vi "cwlaserShutterOpenClose.vi"(1 "mode":u16(ring) items=["close", "open"], 2 "wavelength (nm)":dbl) -> (0 "success":bool)   [LabVIEW 2017]
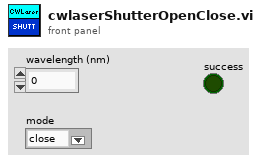
[diagram p1: front panel]
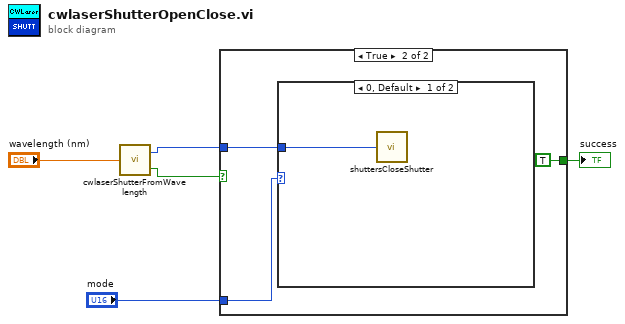
[diagram p0: block diagram]
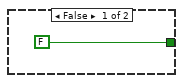
[diagram p2: hidden frame]
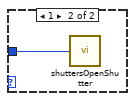
[diagram p3: hidden frame]
diagram:
  n1 = call "cwlaserShutterFromWavelength.vi"("wavelength (nm)"="wavelength (nm)") -> ("shutter"=w3:i32, "found"=w2:bool)
  n2 = case shown="True" w2 {
    tunnel: w3 -> [_ w8]
    tunnel: "mode" -> [_ w9]
    tunnel: [FALSE TRUE] -> w4
    frame False {
    }
    frame True {
      n3 = case shown="0, Default" w9 {
        tunnel: w8 -> [w10 w11]
        frame 0, Default {
          n4 = call "shuttersCloseShutter.vi"("shutter"=w10) -> ()  [unwired: 1 in]
        }
        frame 1 {
          n5 = call "shuttersOpenShutter.vi"("shutter"=w11) -> ()  [unwired: 1 in]
        }
      }
    }
  }
  "success" <- w4
